vi "CMYK to RGB.vi"(0 "Cyan(%)":dbl format="%#.2g", 5 "Magenta(%)":dbl format="%#.2g", 7 "Yellow(%)":dbl format="%#.2g", 9 "Key/Black(%)":dbl format="%#.2g", 11 "error in (no error)":errorcluster) -> (4 "Red":u8, 6 "Green":u8, 8 "Blue":u8, 15 "error out":errorcluster)   [LabVIEW 2018, in "Colour Lab.lvlib"]
uses:
  Colour Lab.lvlib
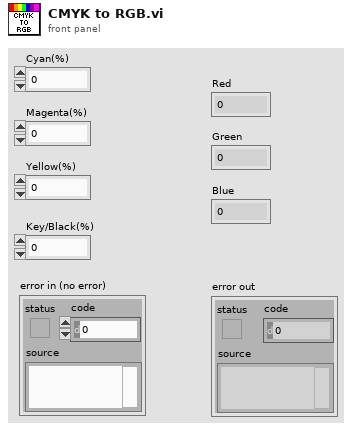
[diagram p1: front panel]
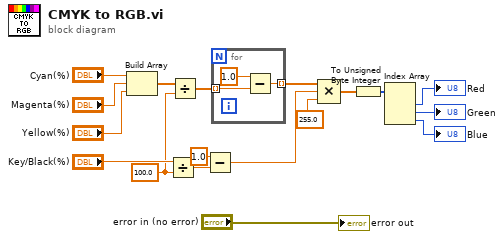
[diagram p0: block diagram]
diagram:
  w5 = 100.0
  n1 = Build Array("Cyan(%)", "Magenta(%)", "Yellow(%)") -> (w15:dbl[])
  n2 = Divide(x="Key/Black(%)", y=w5) -> (x/y=w9:dbl)
  n3 = Divide(x=w15, y=w5) -> (x/y=w4:dbl[])
  n4 = Subtract(x=1.0, y=w9) -> (x-y=w6:dbl)
  n5 = for {
    tunnel: w4 -> [w21] mode=indexing
    tunnel: [w19] -> w3 mode=indexing
    n6 = Subtract(x=1.0, y=w21) -> (x-y=w19:dbl)
  }
  n7 = Compound Arithmetic op=MULTIPLY(w3, w6, 255.0) -> (w1:dbl[])
  n8 = To Unsigned Byte Integer(number=w1) -> (unsigned 8bit integer=w2:u8[])
  n9 = Index Array(array=w2) -> (element #1=→"Red":u8, element #2=→"Green":u8, element #3=→"Blue":u8)  [unwired: 3 in]
  "error out" <- "error in (no error)"
